vi "niSwitch Get Relay Position Wrapper.vi"(8 "error in":errorcluster, 10 "relay name":string, 11 "session factory in":refnum<class "Session Factory.lvclass">) -> (0 "error out":errorcluster, 2 "position":T1=10 items=["Open"=10, "Closed"=11], 3 "session factory out":refnum<class "Session Factory.lvclass">)   [LabVIEW 2021, in "Session Management niSwitch.lvlib" / "Session Factory.lvclass"]
doc: "Returns the relay position for the relay specified in <B>relay name</B>."
uses:
  Session Factory.lvclass
  <instrlib>/niSwitch/niSwitch.llb/niSwitch Relay Position.ctl
  NI Switch_client/RPC Messages/niswitch_grpc_GetRelayPositionRequest.ctl
  NI Switch_client/RPC Messages/nidevice_grpc_Session.ctl
  NI Switch_client/RPC Messages/nidevice_grpc_Session_session/nidevice_grpc_Session_session.lvclass
  Session Factory.lvclass/Session Factory.ctl
  NI Switch_client/NI Switch_client.lvlib
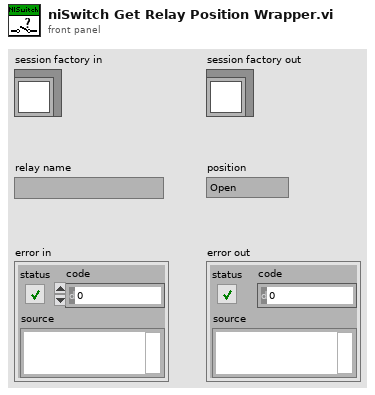
[diagram p1: front panel]
types:
  T1 = typedef "niSwitch Relay Position.ctl" = i32
  T2 = typedef "NI Switch_client.lvlib/niswitch_grpc_GetRelayPositionRequest.ctl" = cluster{"vi":T3, "relay_name":string}
  T3 = typedef "NI Switch_client.lvlib/nidevice_grpc_Session.ctl" = cluster{"nidevice_grpc_Session_session":refnum<class "nidevice_grpc_Session_session.lvclass">}
  T4 = typedef "grpc-lvsupport-release.lvlib/grpcId.ctl" = u64
  T5 = typedef "NI Switch_client.lvlib/niswitch_grpc_GetRelayPositionResponse.ctl" = cluster{"status":i32, "relay_position":T6, "relay_position_raw":i32}
  T6 = typedef "NI Switch_client.lvlib/niswitch_grpc_RelayPosition.ctl" = enum32{"RELAY_POSITION_UNSPECIFIED", "RELAY_POSITION_NISWITCH_VAL_OPEN", "RELAY_POSITION_NISWITCH_VAL_CLOSED"}
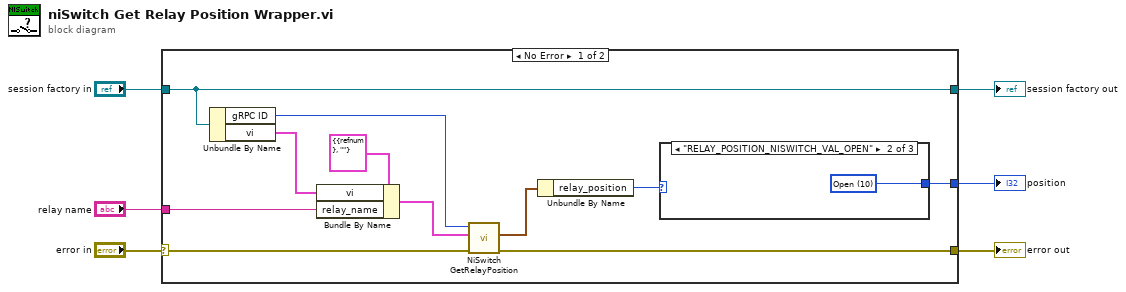
[diagram p0: block diagram]
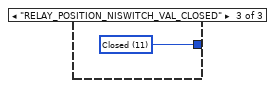
[diagram p3: hidden frame]
diagram:
  n1 = case shown="No Error" "error in" {
    selector: "error in" -> [w14 w20]
    tunnel: [w7 w21] -> w6
    tunnel: "session factory in" -> [w7 w21]
    tunnel: [w10 w20] -> w5
    tunnel: [w13 _] -> w2
    tunnel: "relay name" -> [w8 _]
    frame No Error {
      n2 = Unbundle By Name(w7) -> ("gRPC ID"=w17:T4, "vi"=w15:T3)
      n3 = Bundle By Name(cluster=T2 {"vi"={"nidevice_grpc_Session_session"=refnum}, "relay_name"=""} ("Request Data"), "vi"=w15, "relay_name"=w8) -> (w16:T2)
      n4 = call "NiSwitch GetRelayPosition.vi"("error in"=w14, "Request Data"=w16, "gRPC ID"=w17) -> ("error out"=w10:errorcluster, "Response Data"=w12:T5)  [unwired: 6 in, 1 out]
      n5 = Unbundle By Name(w12) -> ("relay_position"=w11:T6)
      n6 = case shown="\"RELAY_POSITION_NISWITCH_VAL_OPEN\"" w11 {
        tunnel: [_ w18 w19] -> w13
        frame "RELAY_POSITION_UNSPECIFIED", Default {
        }
        frame "RELAY_POSITION_NISWITCH_VAL_OPEN" {
          w18 = T1 10 items=["Open"=10, "Closed"=11] ("position")
        }
        frame "RELAY_POSITION_NISWITCH_VAL_CLOSED" {
          w19 = T1 11 items=["Open"=10, "Closed"=11] ("position")
        }
      }
    }
    frame Error {
    }
  }
  "error out" <- w5
  "session factory out" <- w6
  "position" <- w2
